vi "LNLS Control FOFB Config FOFBC.vi"(8 "error in (no error)":errorcluster, 11 "LNLS Control FOFB Configuration Out":T1={"Status"=0, "Operation Mode"=enum."Manual Mode", "Horizontal Gain"=0.0, "Vertical Gain"=0.0, "Selected Reference Orbit"=0, "Selected Correction Matrix"=0, "Selected FPGA Filters"=0, "Horizontal Distortion Threshold"=0.0, "Vertical Distortion Threshold"=0.0, "Timestamp"=0.0}) -> (0 "error out":errorcluster, 3 "PFOFBC Data":T1={"Status"=0, "Operation Mode"=enum."Manual Mode", "Horizontal Gain"=0.0, "Vertical Gain"=0.0, "Selected Reference Orbit"=0, "Selected Correction Matrix"=0, "Selected FPGA Filters"=0, "Horizontal Distortion Threshold"=0.0, "Vertical Distortion Threshold"=0.0, "Timestamp"=0.0})   [LabVIEW 2011, in "LNLS Control VIs.lvlib"]
uses:
  LNLS Control VIs.lvlib
  Types Definitions/Type Control FOFB Configuration Out.ctl
  Types Definitions/Type Operation Mode State.ctl
  Type Definitions.lvlib
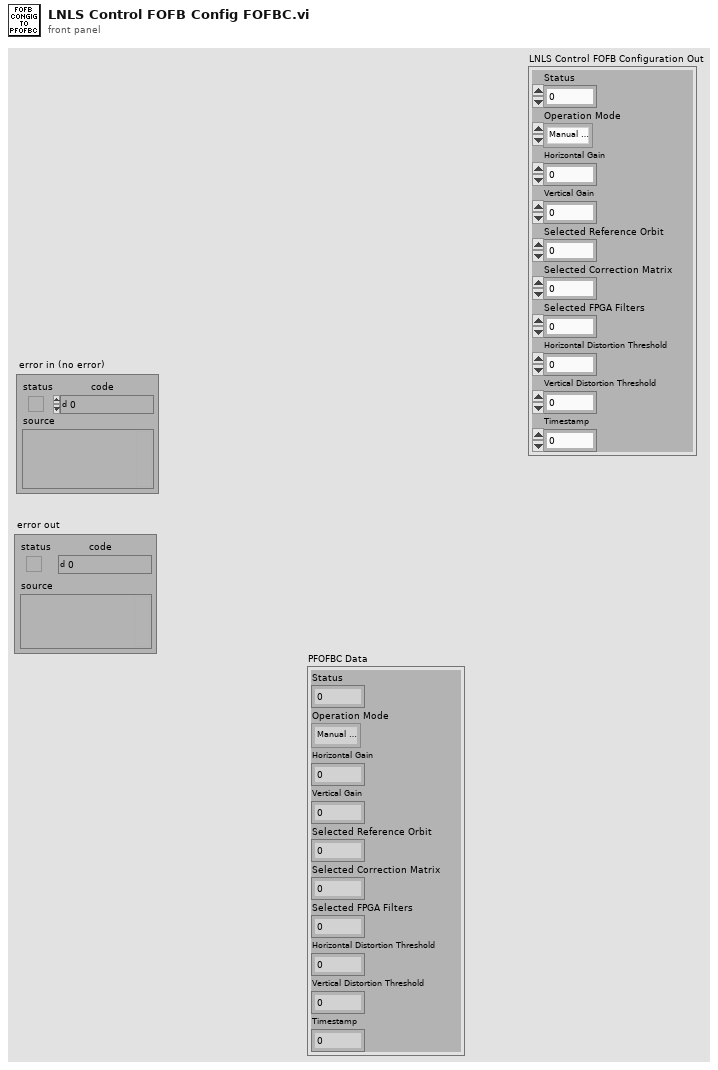
[diagram p1: front panel]
types:
  T1 = typedef "Type Definitions.lvlib/Type Control FOFB Configuration Out.ctl" = cluster{"Status":u16, "Operation Mode":T2, "Horizontal Gain":sgl, "Vertical Gain":sgl, "Selected Reference Orbit":i32, "Selected Correction Matrix":i32, "Selected FPGA Filters":i32, "Horizontal Distortion Threshold":sgl, "Vertical Distortion Threshold":sgl, "Timestamp":dbl}
  T2 = typedef "Type Definitions.lvlib/Type Operation Mode State.ctl" = enum8{"Idle Mode", "Manual Mode", "FOFB Mode"}
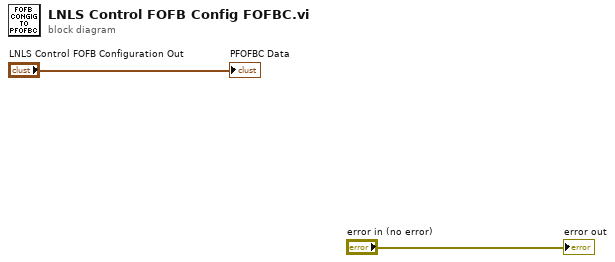
[diagram p0: block diagram]
diagram:
  "error out" <- "error in (no error)"
  "PFOFBC Data" <- "LNLS Control FOFB Configuration Out"
